vi "GetProcessFullName.vi"(8 "error in":errorcluster, 11 "OperationCycle in":refnum<class "OperationCycle.lvclass">) -> (0 "error out":errorcluster, 2 "ProcessFullName":string, 3 "OperationCycle out":refnum<class "OperationCycle.lvclass">)   [LabVIEW 2021, in "ProligentXMLGenerator.lvlib" / "OperationCycle.lvclass"]
doc: "Defines the name of the current process in which this operation cycle is defined. This may be different from the 'ProcessFullName' of the parent 'TopProcessRun' if the current operation is in a sub-process of the top parent.\n\nThis attribute cannot be updated."
uses:
  OperationCycle.lvclass
  OperationCycle.lvclass/OperationCycle.ctl
  Base/ProcessFullName/ProcessFullName.lvclass
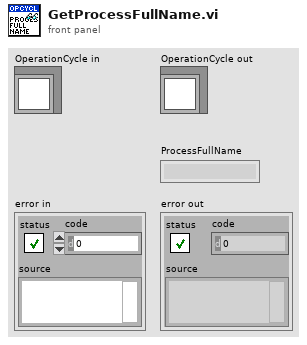
[diagram p1: front panel]
types:
  T1 = typedef "ProligentXMLGenerator.lvlib/OperationCycle.lvclass/Data.ctl" = cluster{"Name":string, "CustomData":refnum<class "CustomData.lvclass">, "ProcessFullName":refnum<class "ProcessFullName.lvclass">, "ProcessVersion":refnum<class "NonEmptyString_64.lvclass">, "OperationCycleId":refnum<class "Guid.lvclass">, "OperationName":refnum<class "NonEmptyString_65.lvclass">, "Location":refnum<class "FullName.lvclass">, "User":refnum<class "NonEmptyString_255.lvclass">, "OperationCycleStatus":refnum<class "ExecutionStatus.lvclass">, "OperationCycleStartTime":refnum<class "DateTime.lvclass">, "OperationCycleEndTime":refnum<class "DateTime.lvclass">, "TimeZoneInfoId":string}
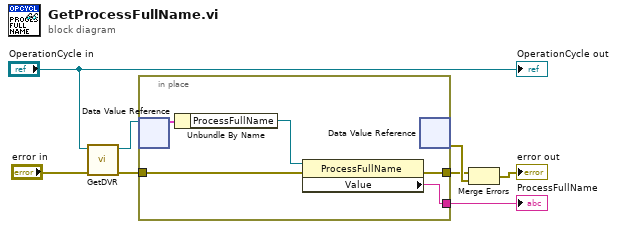
[diagram p0: block diagram]
diagram:
  n1 = call "GetDVR.vi"("error in"="error in", "OperationCycle in"="OperationCycle in") -> ("error out"=w2:errorcluster, "DVRReference"=w7:refnum<data-value>)  [unwired: 8 in]
  n2 = in-place "In Place Element Structure" {
    in-place-border: [w10] -> w6
    in-place-border: w2 -> [w11]
    in-place-border: [w9] -> w1
    n3 = in-place-dvr #1(w7) -> (w13:T1)  [unwired: 1 out]
    n4 = Unbundle By Name(w13) -> ("ProcessFullName"=w12:refnum<class "ProcessFullName.lvclass">)
    n5 = property on="Property Node" class="ProcessFullName"(reference=w12, error in=w11) -> (error out=w9:errorcluster, "Value"=w10:string)  [unwired: 1 out]
    n6 = in-place-dvr #1() -> (w8:errorcluster)  [unwired: 1 in, 1 out]
  }
  "ProcessFullName" <- w6
  n7 = Merge Errors(w1, w8) -> (→"error out":errorcluster)
  "OperationCycle out" <- "OperationCycle in"
